vi "LEBITVacuum.FileTo2dArray.vi"(1 "file path (dialog if empty)":path, 4 "Create if ness.":bool, 5 "error in":errorcluster) -> (17 "Array":string[][](array[string]), 19 "error out":errorcluster)   [LabVIEW 2014, in "LEBITVacuum.lvlib"]
uses:
  LEBITVacuum.lvlib
  CSCore/CSSystem/CoreDefs/CoreDefs.error_type.ctl
  CSCore/CSSystem/CoreDefs/CoreDefs.error_severity.ctl
  CSCore/CSSystem/CoreLib/CoreLib.lvlib
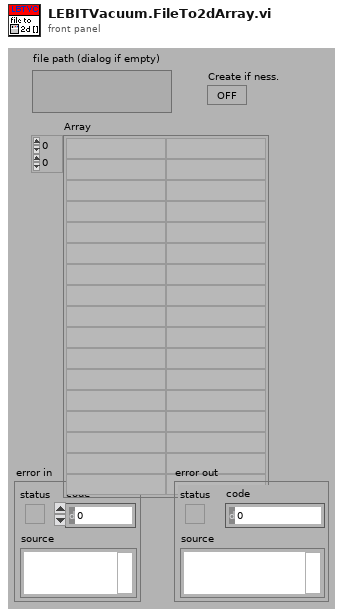
[diagram p1: front panel]
types:
  T1 = typedef "CoreDefs.error_severity.ctl" = enum16{"undefined", "information", "warning", "error", "fatal"}
  T2 = typedef "CoreDefs.error_type.ctl" = enum16{"no error", "can't load process", "can't unload process", "process does not exist", "can't install process", "can't remove process", "unknown function", "time out", "can't execute function", "duplicate queue name", "super not found", "caller queue invalid", "can't ping process", "unknown error", "VISA Error", "VISA timeout", "GPIB timeout", "GPIB error", "communication error", "data type mismatch", "can't read data from OPC server", "can't write data to OPC server", "OET error", "function not implemented", "process already exists", "invalid Shared Variable name", "error writing Shared Variable", "error reading Shared Variable", "invalid client name", "corrupt database", "unknown class", "call not authorized", "parameter out of range", "OET timeout: can't get data to modify", "invalid queue name", "requested operation incompatible with current state", "event undefined", "event disabled", "state undefined", "caller is not a friend", "EventBuilder: bad eventID", "EventBuilder: no DAQ devices", "a thread must not stop itself", "UNUSED ELEMENT4", "DiscArchiver: eventData incomplete", "DiscArchiver: eventData does not belong to run", "DiscArchiver: can't open file", "DiscArchiver: can't write to file", "DiscArchiver: available disc space low", "can't acquire semaphore", "error reading data from database", "notifier object is not existing", "can't register process", "can't unregister process", "illegal event type", "object disabled", "object already exists", "can't change state", "Instrument not found", "no connection to remote node", "invalid reference", "N/A", "UNUSED ELEMENT 1", "element not found", "illegal TCP/IP connection detected", "object does not exist", "invalid access ID", "unknown CS system", "invalid privilige", "unsupported data type", "unsupported server type", "IO server already exists", "Shared Variable already exists"}
  T3 = enum16{"open", "replace", "create", "open or create", "replace or create", "replace or create with confirmation"}
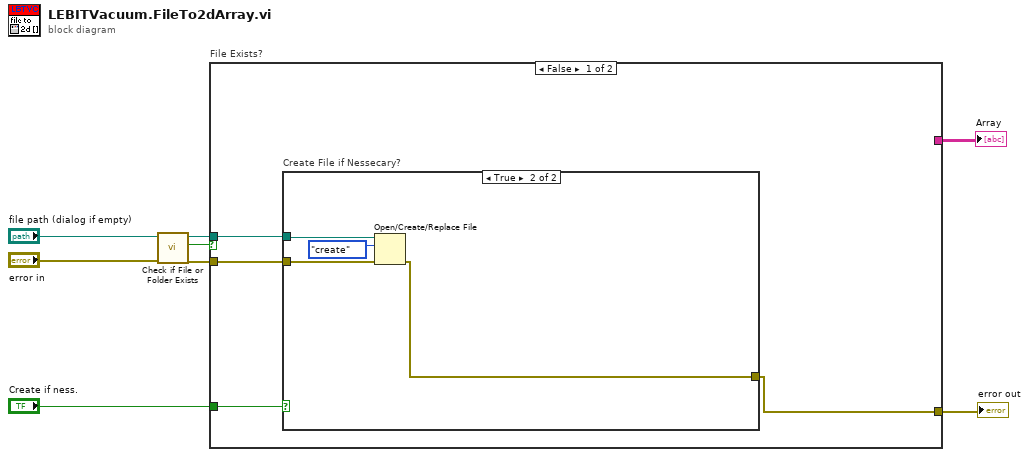
[diagram p0: block diagram]
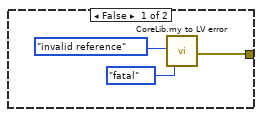
[diagram p2: hidden frame]
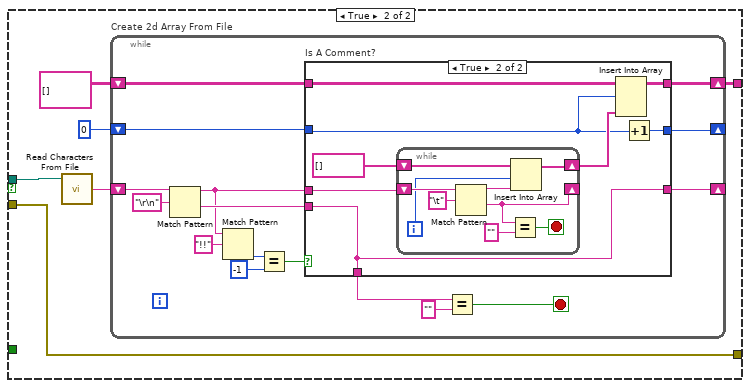
[diagram p3: hidden frame]
diagram:
  n1 = call <vilib>:"Check if File or Folder Exists.vi"("error in (no error)"="error in", "path"="file path (dialog if empty)") -> ("error out"=w6:errorcluster, "file or folder exists?"=w7:bool, "dup path"=w8:path)  [unwired: 7 in]
  n2 = case "File Exists?" shown="False" w7 {
    tunnel: w8 -> [w12 w23]
    tunnel: [_ w22] -> w2
    tunnel: w6 -> [w11 w21]
    tunnel: [w10 w21] -> w1
    tunnel: "Create if ness." -> [w9 _]
    frame False {
      n3 = case "Create File if Nessecary?" shown="True" w9 {
        tunnel: w12 -> [_ w18]
        tunnel: w11 -> [_ w17]
        tunnel: [w13 w16] -> w10
        frame False {
          n4 = call "CoreLib.my to LV error.vi"("ErrorTypes"=CoreDefs.error_type."invalid reference", "severityLevel"=CoreDefs.error_severity."fatal") -> ("myErrorCluster"=w13:errorcluster)  [unwired: 16 in, 1 out]
        }
        frame True {
          n5 = Open/Create/Replace File(file path (use dialog)=w18, error in=w17, operation (0:open)=T3."create") -> (error out=w16:errorcluster)  [unwired: 3 in, 2 out]
        }
      }
    }
    frame True {
      n6 = call <vilib>:"Read Characters From File.vi"("file path (dialog if empty)"=w23) -> ("character string"=w25:string)  [unwired: 5 in, 3 out]
      n7 = while "Create 2d Array From File" {
        shift-right: [w31] -> _
        shift-left: w25 -> [w41]
        shift-right: [w39] -> w22
        shift-left: string[][] [] -> [w38]
        shift-right: [w29] -> _
        shift-left: 0 -> [w30]
        stop <- w27 stop-if-true
        n8 = Match Pattern(string=w41, regular expression="\r\n") -> (before substring=w36:string, after substring=w37:string)  [unwired: 1 in, 2 out]
        n9 = Match Pattern(string=w36, regular expression="!!") -> (offset past match=w34:i32)  [unwired: 1 in, 3 out]
        n10 = Equal?(x=w34, y=-1) -> (x = y?=w32:bool)
        n11 = case "Is A Comment?" shown="True" w32 {
          tunnel: [w43 w51] -> w39
          tunnel: w38 -> [w43 w50]
          tunnel: w37 -> [w42 w45]
          tunnel: w36 -> [_ w48]
          tunnel: [w42 w45] -> w31
          tunnel: w30 -> [w44 w47]
          tunnel: [w44 w46] -> w29
          tunnel: [w42 w45] -> w26
          frame False {
          }
          frame True {
            n12 = while {
              shift-right: [w55] -> _
              shift-left: w48 -> [w61]
              shift-right: [w56] -> w49
              shift-left: string[] [] -> [w59]
              i -> [w57]
              stop <- w53 stop-if-true
              n13 = Match Pattern(string=w61, regular expression="\t") -> (before substring=w58:string, after substring=w55:string)  [unwired: 1 in, 2 out]
              n14 = Equal?(x=w55, y="") -> (x = y?=w53:bool)
              n15 = Insert Into Array(array=w59, index=w57, new element=w58) -> (w56:string[])
            }
            n16 = Insert Into Array(array=w50, index (row)=w47, new element=w49) -> (w51:string[][])  [unwired: 1 in]
            n17 = Increment(x=w47) -> (x+1=w46:i32)
          }
        }
        n18 = Equal?(x=w26, y="") -> (x = y?=w27:bool)
      }
    }
  }
  "Array" <- w2
  "error out" <- w1
